vi "CurrentTime.vi"(8 "error in":errorcluster caption="错误输入（无错误）", 11 "Input1":T1) -> (0 "error out":errorcluster caption="错误输出")   [LabVIEW 2013]
uses:
  Input1.ctl
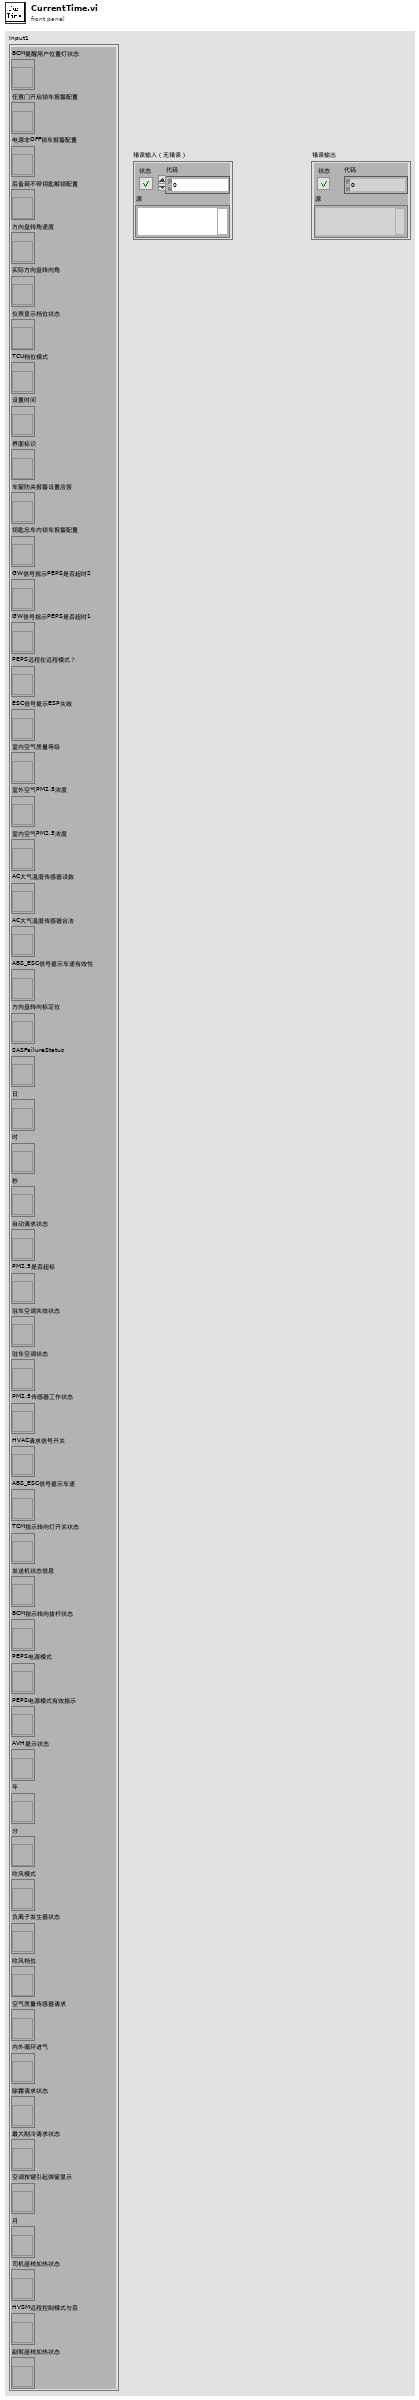
[diagram p1: front panel]
types:
  T1 = typedef "Input1.ctl" = cluster{"BCM提醒用户位置灯状态":refnum<vi>, "任意门开启锁车报警配置":refnum<vi>, "电源非OFF锁车报警配置":refnum<vi>, "后备箱不带钥匙解锁配置":refnum<vi>, "方向盘转角速度":refnum<vi>, "实际方向盘转向角":refnum<vi>, "仪表显示档位状态":refnum<vi>, "TCU档位模式":refnum<vi>, "设置时间":refnum<vi>, "界面标识":refnum<vi>, "车窗防夹报警设置应答":refnum<vi>, "钥匙忘车内锁车报警配置":refnum<vi>, "GW信号指示PEPS是否超时2":refnum<vi>, "GW信号指示PEPS是否超时1":refnum<vi>, "PEPS远程在远程模式？":refnum<vi>, "ESC信号提示ESP失败":refnum<vi>, "室内空气质量等级":refnum<vi>, "室外空气PM2.5浓度":refnum<vi>, "室内空气PM2.5浓度":refnum<vi>, "AC大气温度传感器读数":refnum<vi>, "AC大气温度传感器合法":refnum<vi>, "ABS_ESC信号提示车速有效性":refnum<vi>, "方向盘转向标定位":refnum<vi>, "SASFailureStatus":refnum<vi>, "日":refnum<vi>, "时":refnum<vi>, "秒":refnum<vi>, "自动请求状态":refnum<vi>, "PM2.5是否超标":refnum<vi>, "驻车空调失效状态":refnum<vi>, "驻车空调状态":refnum<vi>, "PM2.5传感器工作状态":refnum<vi>, "HVAC请求信号开关":refnum<vi>, "ABS_ESC信号提示车速":refnum<vi>, "TCM指示转向灯开关状态":refnum<vi>, "发送机状态信息":refnum<vi>, "BCM指示转向拔杆状态":refnum<vi>, "PEPS电源模式":refnum<vi>, "PEPS电源模式有效指示":refnum<vi>, "AVH提示状态":refnum<vi>, "年":refnum<vi>, "分":refnum<vi>, "吹风模式":refnum<vi>, "负离子发生器状态":refnum<vi>, "吹风档位":refnum<vi>, "空气质量传感器请求":refnum<vi>, "内外循环进气":refnum<vi>, "除霜请求状态":refnum<vi>, "最大制冷请求状态":refnum<vi>, "空调按键引起弹窗显示":refnum<vi>, "月":refnum<vi>, "司机座椅加热状态":refnum<vi>, "HVSM远程控制模式与否":refnum<vi>, "副驾座椅加热状态":refnum<vi>}
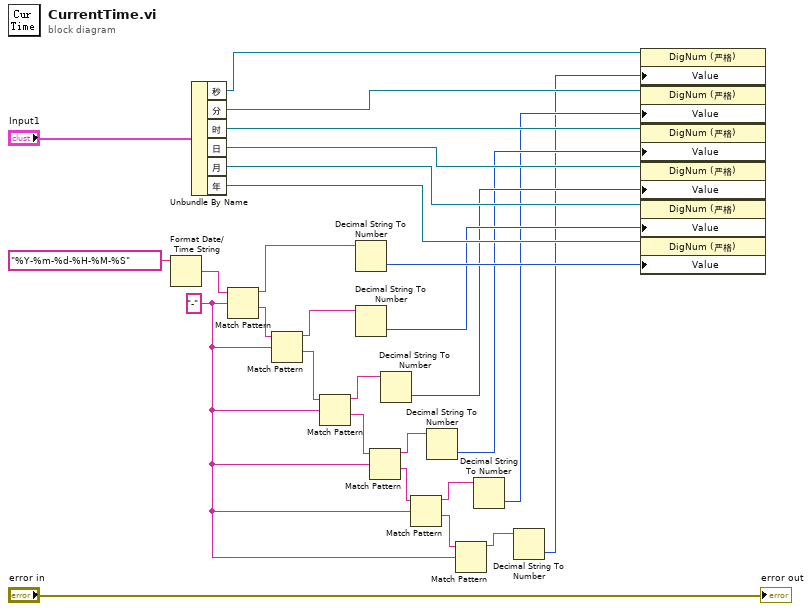
[diagram p0: block diagram]
diagram:
  w20 = "-"
  n1 = Format Date/Time String(time format string (%c)="%Y-%m-%d-%H-%M-%S" ("时间格式字符串(%c)")) -> (date/time string=w26:string)  [unwired: 2 in]
  n2 = Unbundle By Name("Input1") -> ("秒"=w10:refnum<vi>, "分"=w2:refnum<vi>, "时"=w5:refnum<vi>, "日"=w7:refnum<vi>, "月"=w9:refnum<vi>, "年"=w12:refnum<vi>)
  n3 = Match Pattern(string=w26, regular expression=w20) -> (before substring=w19:string, after substring=w25:string)  [unwired: 1 in, 2 out]
  n4 = Match Pattern(string=w25, regular expression=w20) -> (before substring=w18:string, after substring=w24:string)  [unwired: 1 in, 2 out]
  n5 = Match Pattern(string=w24, regular expression=w20) -> (before substring=w17:string, after substring=w23:string)  [unwired: 1 in, 2 out]
  n6 = Decimal String To Number(string=w19) -> (number=w11:i32)  [unwired: 2 in, 1 out]
  n7 = Decimal String To Number(string=w18) -> (number=w8:i32)  [unwired: 2 in, 1 out]
  n8 = Match Pattern(string=w23, regular expression=w20) -> (before substring=w16:string, after substring=w22:string)  [unwired: 1 in, 2 out]
  n9 = Decimal String To Number(string=w17) -> (number=w6:i32)  [unwired: 2 in, 1 out]
  n10 = Match Pattern(string=w22, regular expression=w20) -> (before substring=w15:string, after substring=w21:string)  [unwired: 1 in, 2 out]
  n11 = Decimal String To Number(string=w16) -> (number=w4:i32)  [unwired: 2 in, 1 out]
  n12 = Match Pattern(string=w21, regular expression=w20) -> (before substring=w14:string)  [unwired: 1 in, 3 out]
  n13 = Decimal String To Number(string=w15) -> (number=w3:i32)  [unwired: 2 in, 1 out]
  n14 = Decimal String To Number(string=w14) -> (number=w1:i32)  [unwired: 2 in, 1 out]
  n15 = property class="DigNum (严格)"(reference=w10, "Value"=w1) -> ()  [unwired: 1 in, 2 out]
  n16 = property class="DigNum (严格)"(reference=w2, "Value"=w3) -> ()  [unwired: 1 in, 2 out]
  n17 = property class="DigNum (严格)"(reference=w5, "Value"=w4) -> ()  [unwired: 1 in, 2 out]
  n18 = property class="DigNum (严格)"(reference=w7, "Value"=w6) -> ()  [unwired: 1 in, 2 out]
  n19 = property class="DigNum (严格)"(reference=w9, "Value"=w8) -> ()  [unwired: 1 in, 2 out]
  n20 = property class="DigNum (严格)"(reference=w12, "Value"=w11) -> ()  [unwired: 1 in, 2 out]
  "error out" <- "error in"
